vi "Tanque.vi"() -> ()   [LabVIEW 2014]
panel:
  in  "Hf":dbl
  out "K":dbl
  out "Elapsed Time (s)":dbl
  in  "H0":dbl
  out "Numeric":dbl
  in  "A2":dbl
  in  "A1":dbl
  in  "G":dbl
  out "Tank":dbl(slide) scale=0.0..0.3
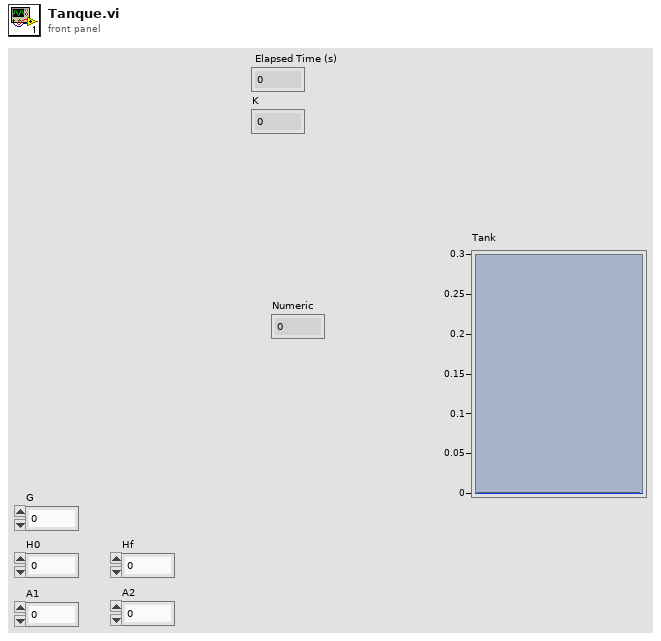
[diagram p1: front panel]
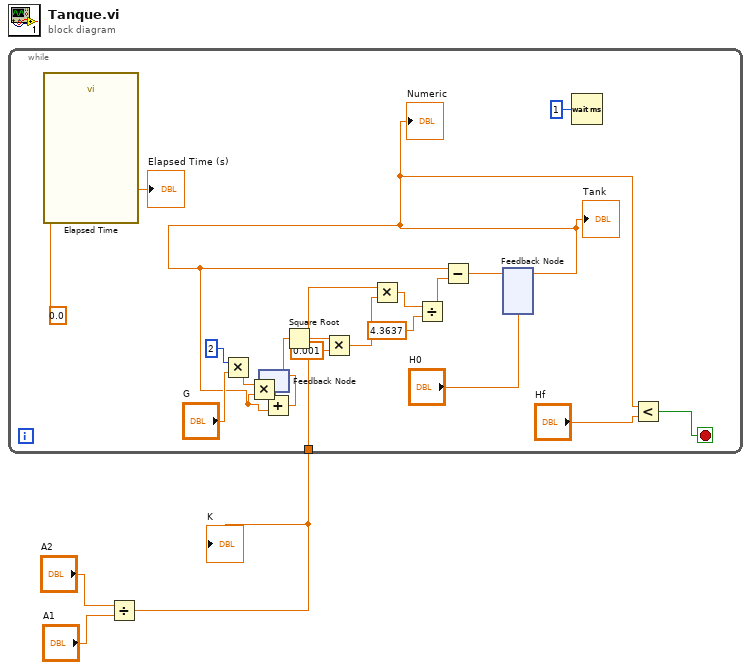
[diagram p0: block diagram]
diagram:
  n1 = Divide(x="A2", y="A1") -> (x/y=w1:dbl)
  "K" <- w1
  n2 = while {
    tunnel: w1 -> [w23]
    stop <- w4 stop-if-true
    n3 = call "Elapsed Time"("Set Start Time (s)"=0.0) -> ("Elapsed Time (s)"=→"Elapsed Time (s)":dbl)  [unwired: 11 in, 7 out]
    n4 = Multiply(x=2, y="G") -> (x*y=w20:dbl)
    n5 = feedback #1() -> (w17:dbl)  [unwired: 1 in]
    n6 = Square Root(x=w17) -> (sqrt(x)=w12:dbl)
    n7 = Multiply(x=w12, y=0.001) -> (x*y=w10:dbl)
    n8 = Multiply(x=w23, y=w10) -> (x*y=w9:dbl)
    n9 = Divide(x=w9, y=4.3637) -> (x/y=w8:dbl)
    n10 = feedback #2("H0") -> (w6:dbl)
    "Tank" <- w6
    "Numeric" <- w6
    n11 = Multiply(x=w20, y=w6) -> (x*y=w19:dbl)
    n12 = Add(x=w19, y=w6) -> (x+y=w18:dbl)
    n13 = feedback-in #1(w18) -> ()
    n14 = Subtract(x=w6, y=w8) -> (x-y=w16:dbl)
    n15 = feedback-in #2(w16) -> ()
    n16 = Wait (ms)(milliseconds to wait=u32 1) -> ()  [unwired: 1 out]
    n17 = Less?(x=w6, y="Hf") -> (x < y?=w4:bool)
  }
